vi "Sub_Kalman_gated.vi"(11 "KF":T2={"State"=[[1.0], [0.0]], "F state prop matrix"=[[1.0, 0.0], [0.0, 1.0]], "H measure matrix"=[[1.0, 0.0]], "P process cov"=[], "R measure cov"=[], "Q state cov"=[], "T Sample"=0.0, "New Measurement"=0.0, "Measurement Variance"=0.0, "State Variance"=0.0, "Threshold"=0.0, "Initialized"=FALSE}) -> (3 "KF":T2={"State"=[[1.0], [0.0]], "F state prop matrix"=[[1.0, 0.0], [0.0, 1.0]], "H measure matrix"=[[1.0, 0.0]], "P process cov"=[], "R measure cov"=[], "Q state cov"=[], "T Sample"=0.0, "New Measurement"=0.0, "Measurement Variance"=0.0, "State Variance"=0.0, "Threshold"=0.0, "Initialized"=FALSE})   [LabVIEW 2021]
uses:
  <vilib>/Analysis/Matrix/Datatypes/RealMatrix.ctl
  <vilib>/Analysis/baseanly.llb/Real A x B.vi
  <vilib>/Analysis/Matrix/Numeric/Add/Add - RM,RM.vi
  <vilib>/Analysis/baseanly.llb/Real Inverse Matrix.vi
  <vilib>/Analysis/Matrix/Numeric/Subtract/Subtract (Elementwise) - RM,R.vi
  <vilib>/Analysis/Matrix/Numeric/Subtract/Subtract - RM,RM.vi
  <vilib>/Analysis/Matrix/NI_Matrix.lvlib
  <vilib>/Analysis/NI_AALBase.lvlib
panel:
  out "x/y":T1
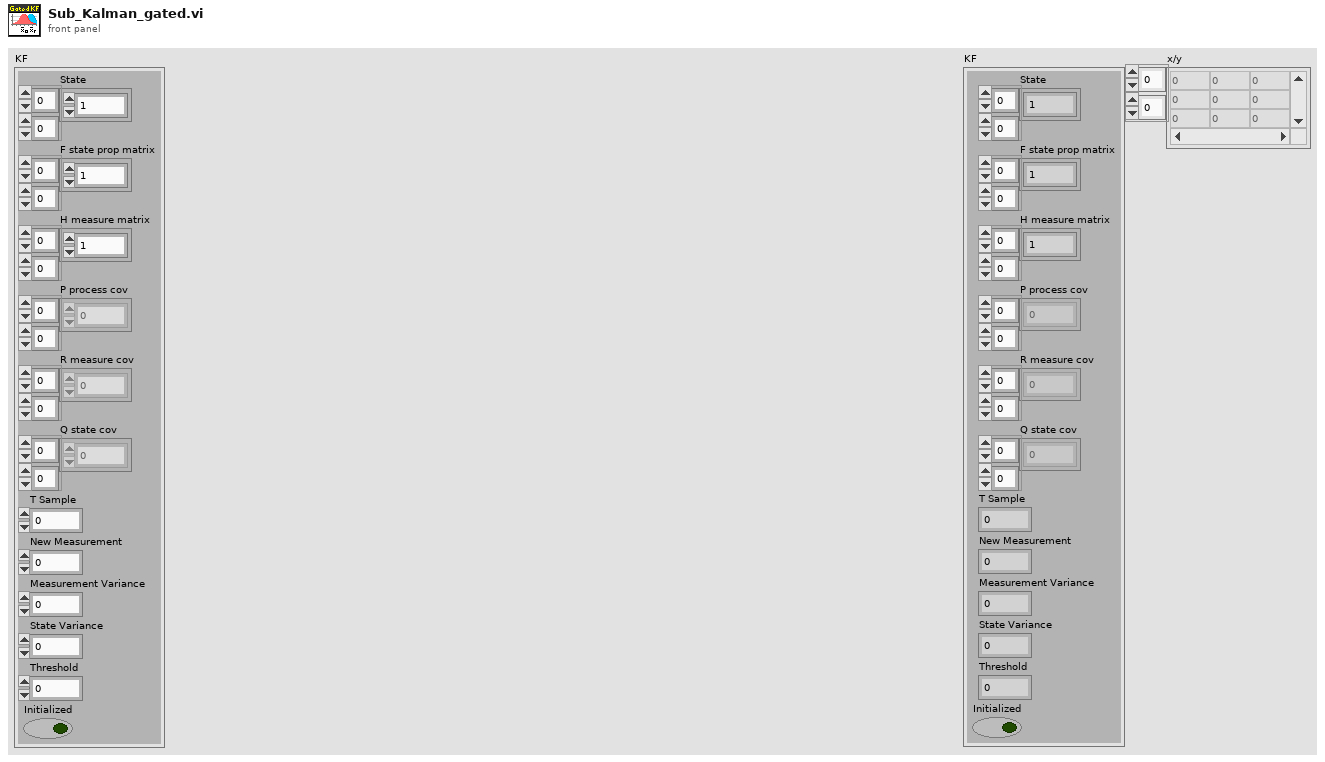
[diagram p1: front panel]
types:
  T1 = typedef "NI_Matrix.lvlib/RealMatrix.ctl" = dbl[][]
  T2 = cluster{"State":dbl[][], "F state prop matrix":dbl[][], "H measure matrix":dbl[][], "P process cov":dbl[][], "R measure cov":dbl[][], "Q state cov":dbl[][], "T Sample":dbl, "New Measurement":dbl, "Measurement Variance":dbl, "State Variance":dbl, "Threshold":dbl, "Initialized":bool}
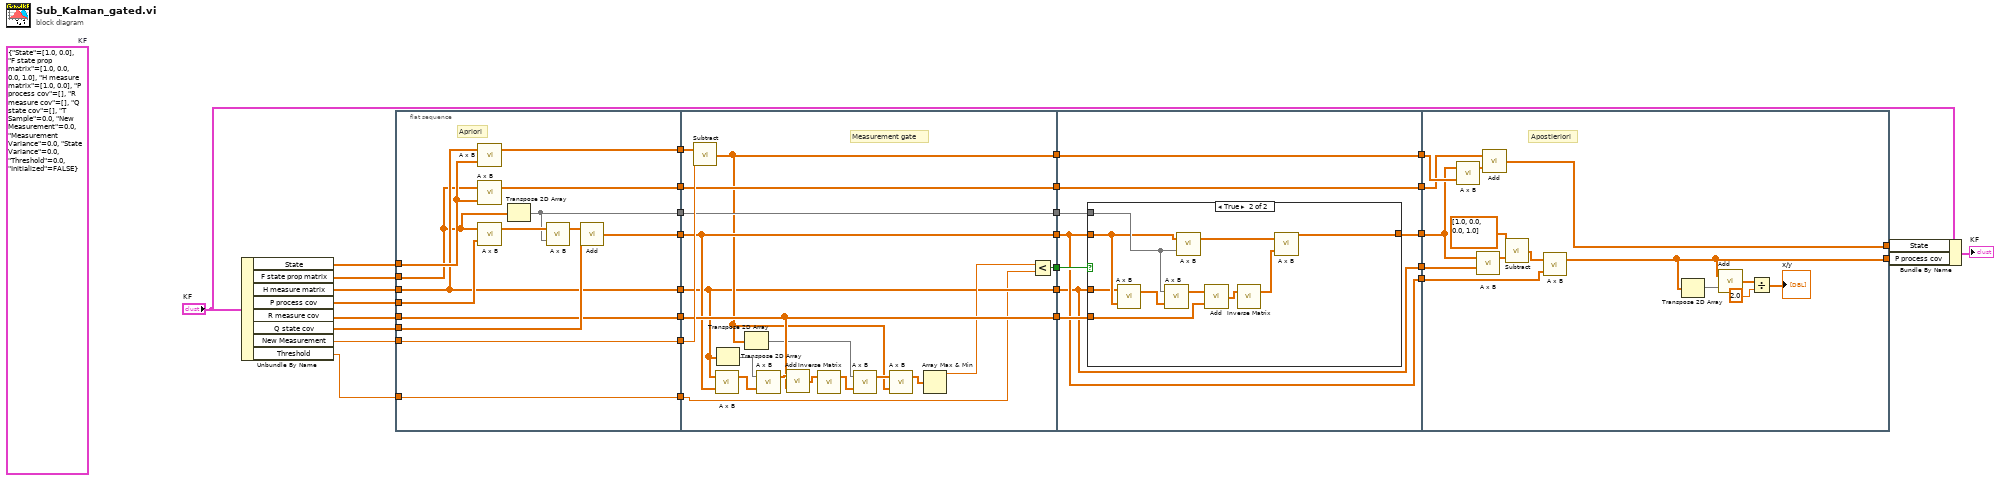
[diagram p0: block diagram]
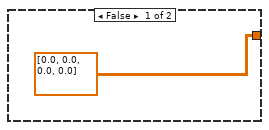
[diagram p2: hidden frame]
diagram:
  (unwired) T2 {"State"=[[1.0], [0.0]], "F state prop matrix"=[[1.0, 0.0], [0.0, 1.0]], "H measure matrix"=[[1.0, 0.0]], "P process cov"=[], "R measure cov"=[], "Q state cov"=[], "T Sample"=0.0, "New Measurement"=0.0, "Measurement Variance"=0.0, "State Variance"=0.0, "Threshold"=0.0, "Initialized"=FALSE}  # KF
  n1 = Unbundle By Name("KF") -> ("State"=w31:dbl[][], "F state prop matrix"=w32:dbl[][], "H measure matrix"=w30:dbl[][], "P process cov"=w26:dbl[][], "R measure cov"=w21:dbl[][], "Q state cov"=w27:dbl[][], "New Measurement"=w20:dbl, "Threshold"=w10:dbl)
  n2 = flat-sequence {
    tunnel: w32 -> [w35]
    tunnel: w31 -> [w42]
    tunnel: w30 -> [w38]
    tunnel: [w46] -> w29
    tunnel: [w45] -> w28
    tunnel: w20 -> [w33]
    tunnel: w27 -> [w44]
    tunnel: w26 -> [w43]
    tunnel: [w39] -> w25
    tunnel: [w34] -> w24
    tunnel: [w38] -> w23
    tunnel: w21 -> [w37]
    tunnel: [w37] -> w22
    tunnel: w10 -> [w36]
    tunnel: [w36] -> w9
    tunnel: [w33] -> w1
    tunnel: w29 -> [w65]
    tunnel: w28 -> [w63]
    tunnel: w25 -> [w55]
    tunnel: [w51] -> w19
    tunnel: w24 -> [w62]
    tunnel: w23 -> [w49]
    tunnel: w22 -> [w59]
    tunnel: [w63] -> w16
    tunnel: [w59] -> w14
    tunnel: [w62] -> w13
    tunnel: [w49] -> w12
    tunnel: [w55] -> w11
    tunnel: w9 -> [w47]
    tunnel: [w52] -> w8
    tunnel: w1 -> [w64]
    tunnel: w19 -> [w73]
    tunnel: [w73] -> w18
    tunnel: [w69] -> w17
    tunnel: w16 -> [w72]
    tunnel: [w72] -> w15
    tunnel: w14 -> [w71]
    tunnel: w13 -> [w70]
    tunnel: w12 -> [w66]
    tunnel: w11 -> [w67]
    tunnel: w8 -> [w68]
    tunnel: [w66] -> w6
    tunnel: [w67] -> w5
    tunnel: w18 -> [w99]
    tunnel: w17 -> [w95]
    tunnel: w15 -> [w97]
    tunnel: [w96] -> w7
    tunnel: w6 -> [w94]
    tunnel: w5 -> [w90]
    tunnel: [w86] -> w2
    frame #0 {
      # "Apriori"
      n3 = call-poly <vilib>:"A x B.vi"("B"=w42, "A"=w38) -> ("A x B"=w46:T1)  [unwired: 1 out]
      n4 = call-poly <vilib>:"A x B.vi"("B"=w42, "A"=w35) -> ("A x B"=w45:T1)  [unwired: 1 out]
      n5 = call-poly <vilib>:"A x B.vi"("B"=w43, "A"=w35) -> ("A x B"=w41:T1)  [unwired: 1 out]
      n6 = Transpose 2D Array(2D array=w35) -> (transposed array=w34:dbl[][])
      n7 = call-poly <vilib>:"A x B.vi"("B"=w34, "A"=w41) -> ("A x B"=w40:T1)  [unwired: 1 out]
      n8 = call-poly <vilib>:"Add.vi"("Real Matrix B"=w44, "Real Matrix A"=w40) -> ("A + B"=w39:T1)
    }
    frame #1 {
      # "Measurement gate"
      n9 = call-poly <vilib>:"Subtract.vi"("Real Scalar c"=w64, "Real Matrix A"=w65) -> ("A - c"=w51:T1)
      n10 = call-poly <vilib>:"A x B.vi"("B"=w55, "A"=w49) -> ("A x B"=w61:T1)  [unwired: 1 out]
      n11 = Transpose 2D Array(2D array=w49) -> (transposed array=w48:dbl[][])
      n12 = Transpose 2D Array(2D array=w51) -> (transposed array=w50:T1)
      n13 = call-poly <vilib>:"A x B.vi"("B"=w61, "A"=w48) -> ("A x B"=w60:T1)  [unwired: 1 out]
      n14 = call-poly <vilib>:"Add.vi"("Real Matrix B"=w59, "Real Matrix A"=w60) -> ("A + B"=w58:T1)
      n15 = call-poly <vilib>:"Inverse Matrix.vi"("Input Matrix"=w58) -> ("Inverse Matrix"=w57:T1)  [unwired: 1 in, 1 out]
      n16 = call-poly <vilib>:"A x B.vi"("B"=w57, "A"=w50) -> ("A x B"=w56:T1)  [unwired: 1 out]
      n17 = call-poly <vilib>:"A x B.vi"("B"=w51, "A"=w56) -> ("A x B"=w54:T1)  [unwired: 1 out]
      n18 = Array Max & Min(array=w54) -> (max value=w53:dbl)  [unwired: 3 out]
      n19 = Less?(x=w53, y=w47) -> (x < y?=w52:bool)
    }
    frame #2 {
      n20 = case shown="True" w68 {
        tunnel: w71 -> [_ w79]
        tunnel: w70 -> [_ w78]
        tunnel: w67 -> [_ w77]
        tunnel: [dbl[][] [[0.0, 0.0], [0.0, 0.0]] w76] -> w69
        tunnel: w66 -> [_ w75]
        frame False {
        }
        frame True {
          n21 = call-poly <vilib>:"A x B.vi"("B"=w77, "A"=w75) -> ("A x B"=w80:T1)  [unwired: 1 out]
          n22 = call-poly <vilib>:"A x B.vi"("B"=w80, "A"=w78) -> ("A x B"=w81:T1)  [unwired: 1 out]
          n23 = call-poly <vilib>:"A x B.vi"("B"=w78, "A"=w77) -> ("A x B"=w82:T1)  [unwired: 1 out]
          n24 = call-poly <vilib>:"Add.vi"("Real Matrix B"=w79, "Real Matrix A"=w81) -> ("A + B"=w83:T1)
          n25 = call-poly <vilib>:"Inverse Matrix.vi"("Input Matrix"=w83) -> ("Inverse Matrix"=w84:T1)  [unwired: 1 in, 1 out]
          n26 = call-poly <vilib>:"A x B.vi"("B"=w84, "A"=w82) -> ("A x B"=w76:T1)  [unwired: 1 out]
        }
      }
    }
    frame #3 {
      # "Apostieriori"
      n27 = call-poly <vilib>:"A x B.vi"("B"=w99, "A"=w95) -> ("A x B"=w98:T1)  [unwired: 1 out]
      n28 = call-poly <vilib>:"A x B.vi"("B"=w94, "A"=w95) -> ("A x B"=w92:T1)  [unwired: 1 out]
      n29 = call-poly <vilib>:"Add.vi"("Real Matrix B"=w98, "Real Matrix A"=w97) -> ("A + B"=w96:T1)
      n30 = call-poly <vilib>:"Subtract.vi"("Real Matrix B"=w92, "Real Matrix A"=dbl[][] [[1.0, 0.0], [0.0, 1.0]]) -> ("A - B"=w91:T1)
      n31 = call-poly <vilib>:"A x B.vi"("B"=w90, "A"=w91) -> ("A x B"=w86:T1)  [unwired: 1 out]
      n32 = Transpose 2D Array(2D array=w86) -> (transposed array=w89:T1)
      n33 = call-poly <vilib>:"Add.vi"("Real Matrix B"=w89, "Real Matrix A"=w86) -> ("A + B"=w88:T1)
      n34 = Divide(x=w88, y=2.0) -> (x/y=→"x/y":T1)
    }
  }
  n35 = Bundle By Name(cluster="KF", "State"=w7, "P process cov"=w2) -> (→"KF":T2)
